vi "TCP Send Data.vi"(6 "error in":errorcluster, 8 "Clients":refnum<k5>[](array[refnum])) -> (0 "error out":errorcluster, 1 "Current Data":dbl, 2 "Clients":refnum<k5>[](array[refnum]), 3 "# of Connections":i32)   [LabVIEW 2020, in "TCP Server.lvlib"]
uses:
  TCP Server.lvlib
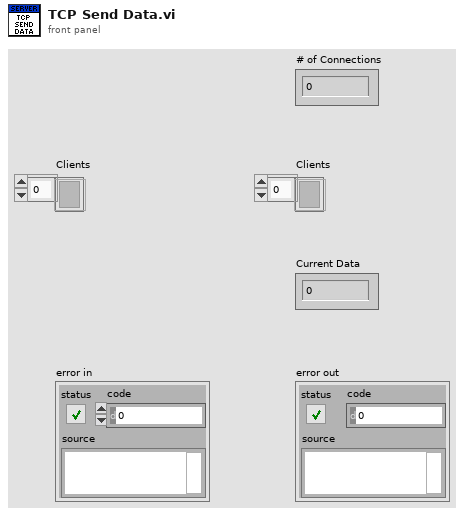
[diagram p1: front panel]
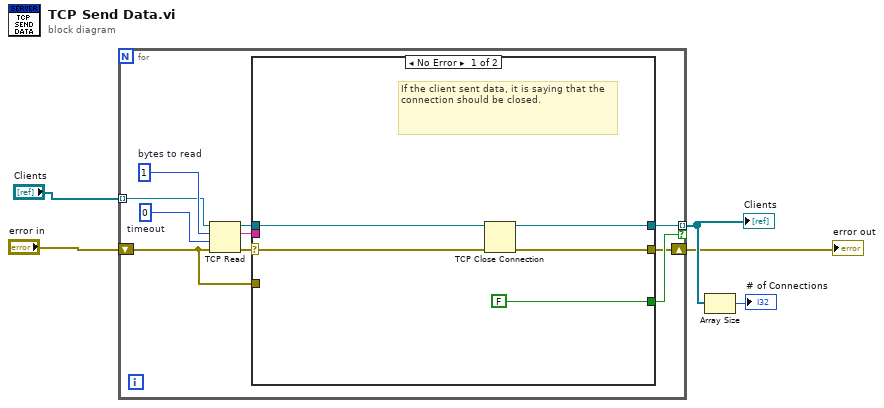
[diagram p0: block diagram]
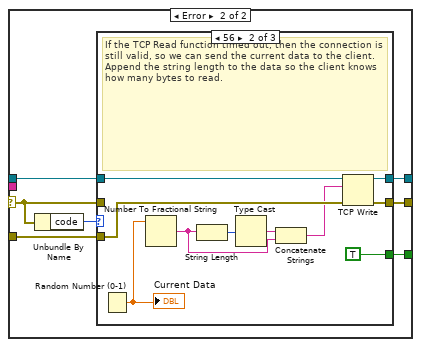
[diagram p2: hidden frame]
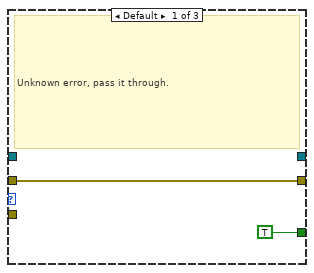
[diagram p3: hidden frame]
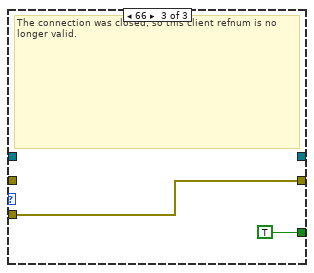
[diagram p4: hidden frame]
diagram:
  n1 = for {
    shift-right: [w8] -> w2
    shift-left: "error in" -> [w7]
    tunnel: [w10] -> w4 mode=indexing if=w9
    tunnel: "Clients" -> [w6] mode=indexing
    w13 = 0  # timeout
    w14 = 1  # bytes to read
    n2 = TCP Read(connection ID=w6, bytes to read=w14, error in (no error)=w7, 9:w13) -> (connection ID out=w15:refnum<k5>, data out=w11:string, error out=w12:errorcluster)  [unwired: 1 out]
    n3 = case shown="No Error" w12 {
      selector: w12 -> [w19 w26]
      tunnel: w15 -> [w20 w23]
      tunnel: w11 -> [_ _]
      tunnel: [w16 w21] -> w10
      tunnel: [FALSE w22] -> w9
      tunnel: [w17 w25] -> w8
      tunnel: w7 -> [_ w24]
      frame No Error {
        # "If the client sent data, it is saying that the connection should be closed."
        # "If the client sent data, it is saying that the connection should be closed."
        n4 = TCP Close Connection(connection ID=w20, error in (no error)=w19) -> (connection ID out=w16:refnum<k5>, error out=w17:errorcluster)  [unwired: 1 out]
      }
      frame Error {
        # "Ignore connection closed and timeout errors"
        n5 = Unbundle By Name(w26) -> ("code"=w27:i32)
        n6 = case shown="56" w27 {
          tunnel: w26 -> [w29 _ _]
          tunnel: [w29 w39 w41] -> w25
          tunnel: w24 -> [_ w35 w41]
          tunnel: w23 -> [_ w38 _]
          tunnel: [TRUE TRUE TRUE] -> w22
          tunnel: [_ w37 _] -> w21
          frame Default {
            # "Unknown error, pass it through."
          }
          frame 56 {
            # "If the TCP Read function timed out, then the connection is still valid, so we can send the current data to the client. Append the string length to the data so the client knows how many bytes to read."
            n7 = Random Number (0-1)() -> (number: 0 to 1=w34:dbl)
            "Current Data" <- w34
            n8 = Number To Fractional String(number=w34) -> (F-format string=w31:string)  [unwired: 3 in]
            n9 = String Length(string=w31) -> (length=w32:i32)
            n10 = Type Cast(x=w32) -> (*(type *) &x=w33:string)  [unwired: 1 in]
            n11 = Concatenate Strings(w33, w31) -> (w30:string)
            n12 = TCP Write(connection ID=w38, data in=w30, error in (no error)=w35) -> (connection ID out=w37:refnum<k5>, error out=w39:errorcluster)  [unwired: 2 out]
          }
          frame 66 {
            # "The connection was closed, so this client refnum is no longer valid."
          }
        }
      }
    }
  }
  "Clients" <- w4
  "error out" <- w2
  n13 = Array Size(array=w4) -> (size(s)=→"# of Connections":i32)
